vi "Folder and Path Creation.vi"(7 "Action":T1, 8 "Error In":errorcluster, 11 "Source Path for Copy":path) -> (0 "Error Out":errorcluster, 2 "Cancelled?":bool, 3 "CSV File path":path)   [LabVIEW 2012]
doc: "Generate the path to store the position save file.\nThe default position in the date folder (where the raw files are also saved)"
uses:
  Folder and Path Creation_Commands.ctl
  <vilib>/Utility/file.llb/Read From Spreadsheet File (string).vi
  <vilib>/Utility/file.llb/Write To Spreadsheet File (string).vi
  GFG/GFG library.lvlib
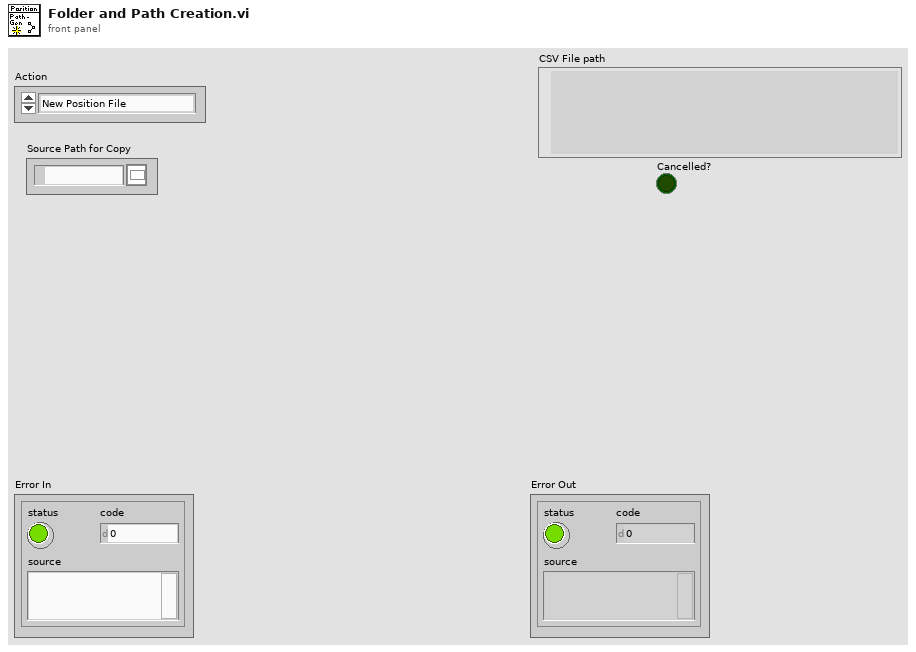
[diagram p1: front panel]
types:
  T1 = typedef "Folder and Path Creation_Commands.ctl" = enum16{"New Position File", "Load Position File", "Copy Position File"}
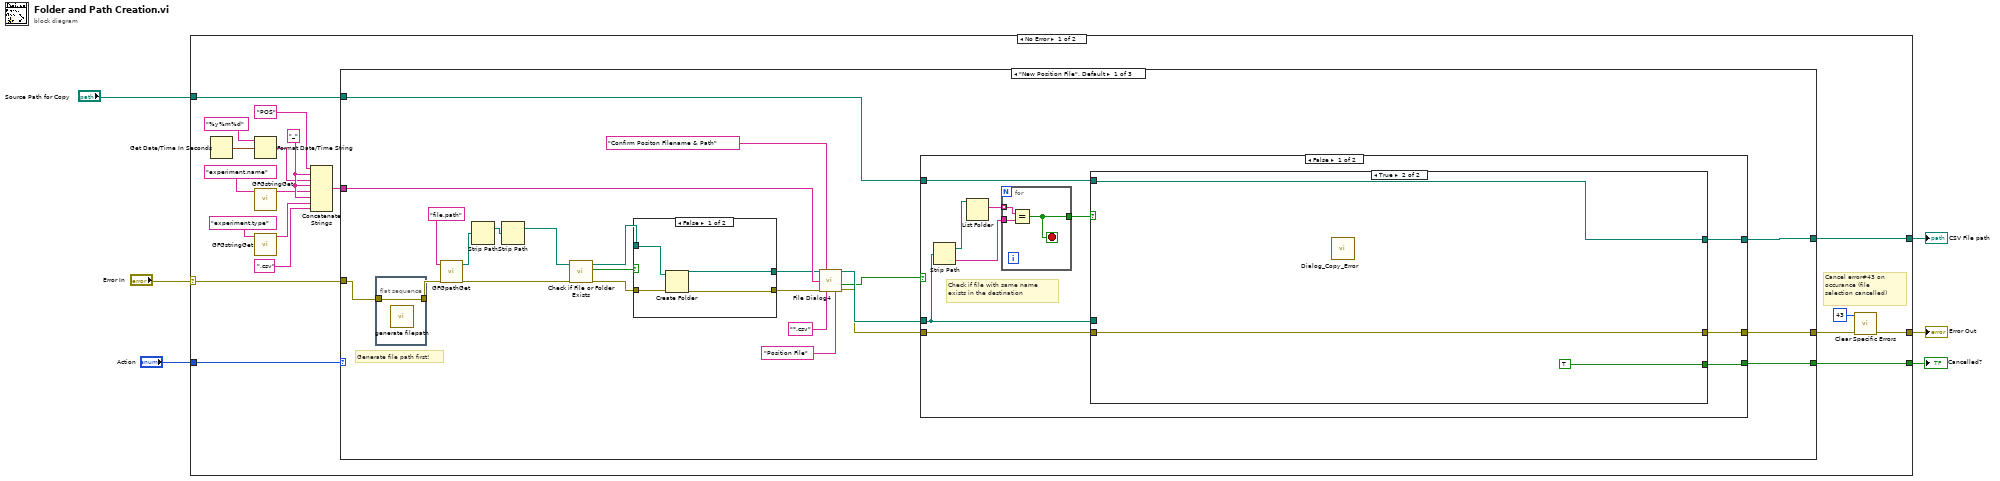
[diagram p0: block diagram]
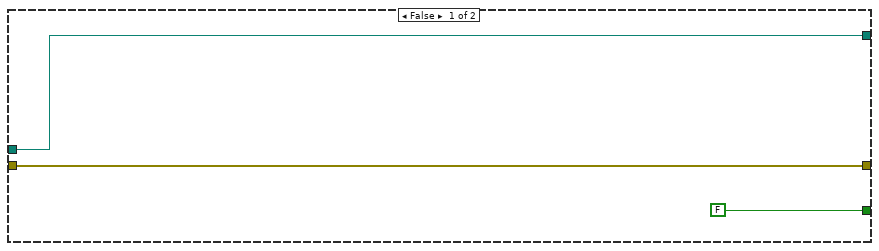
[diagram p2: hidden frame]
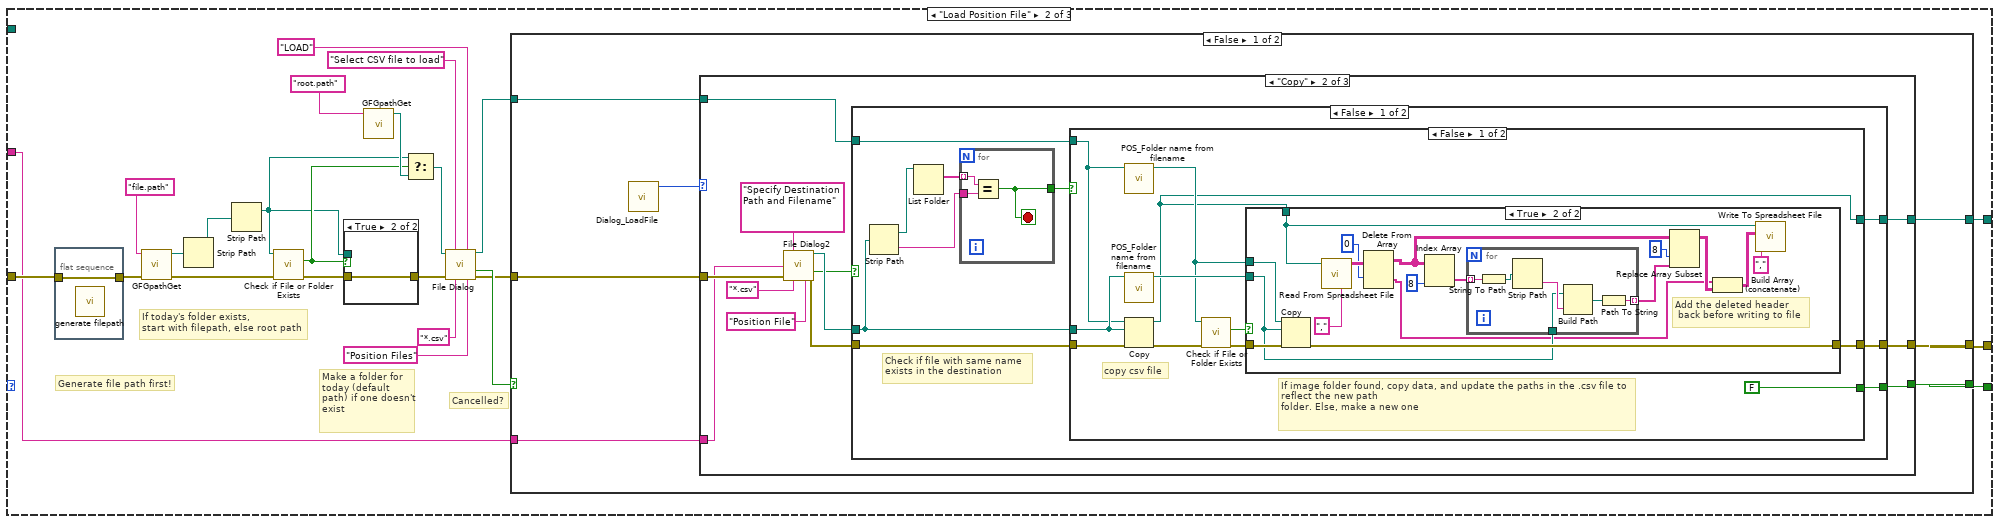
[diagram p5: hidden frame]
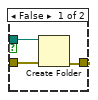
[diagram p6: hidden frame]
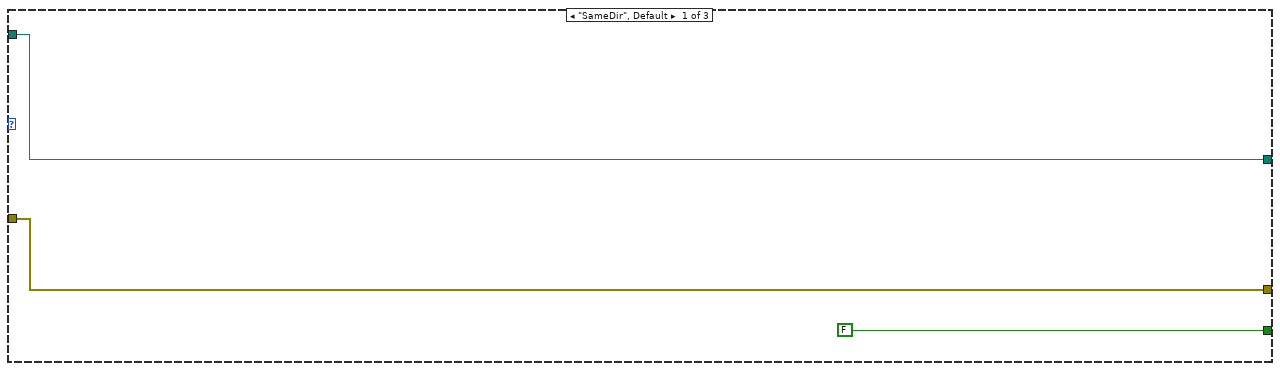
[diagram p7: hidden frame]
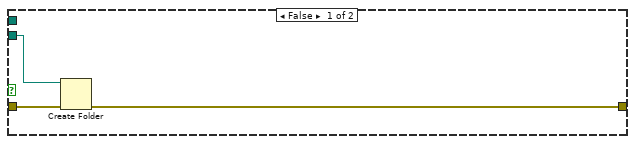
[diagram p8: hidden frame]
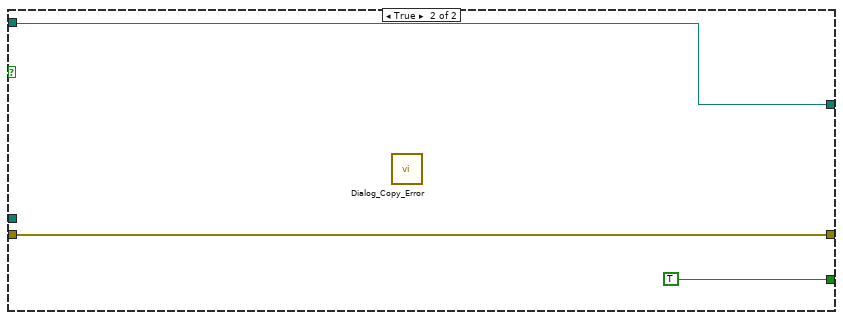
[diagram p9: hidden frame]
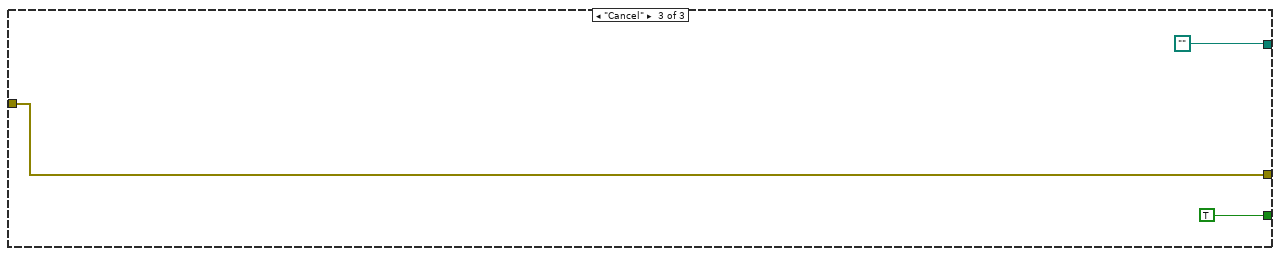
[diagram p11: hidden frame]
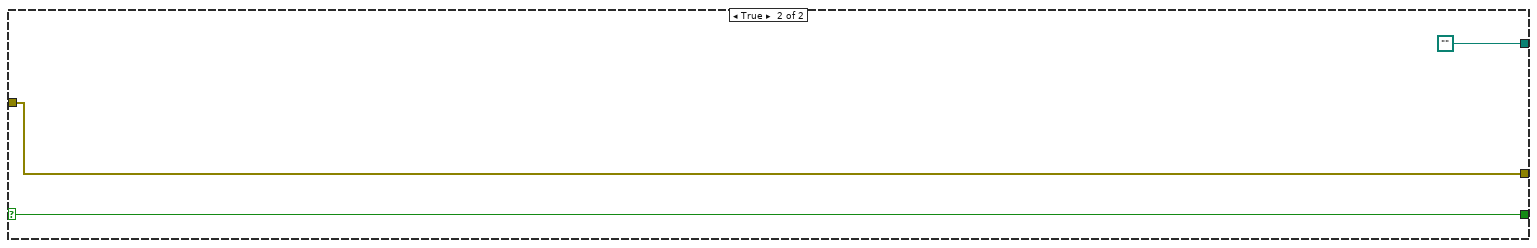
[diagram p12: hidden frame]
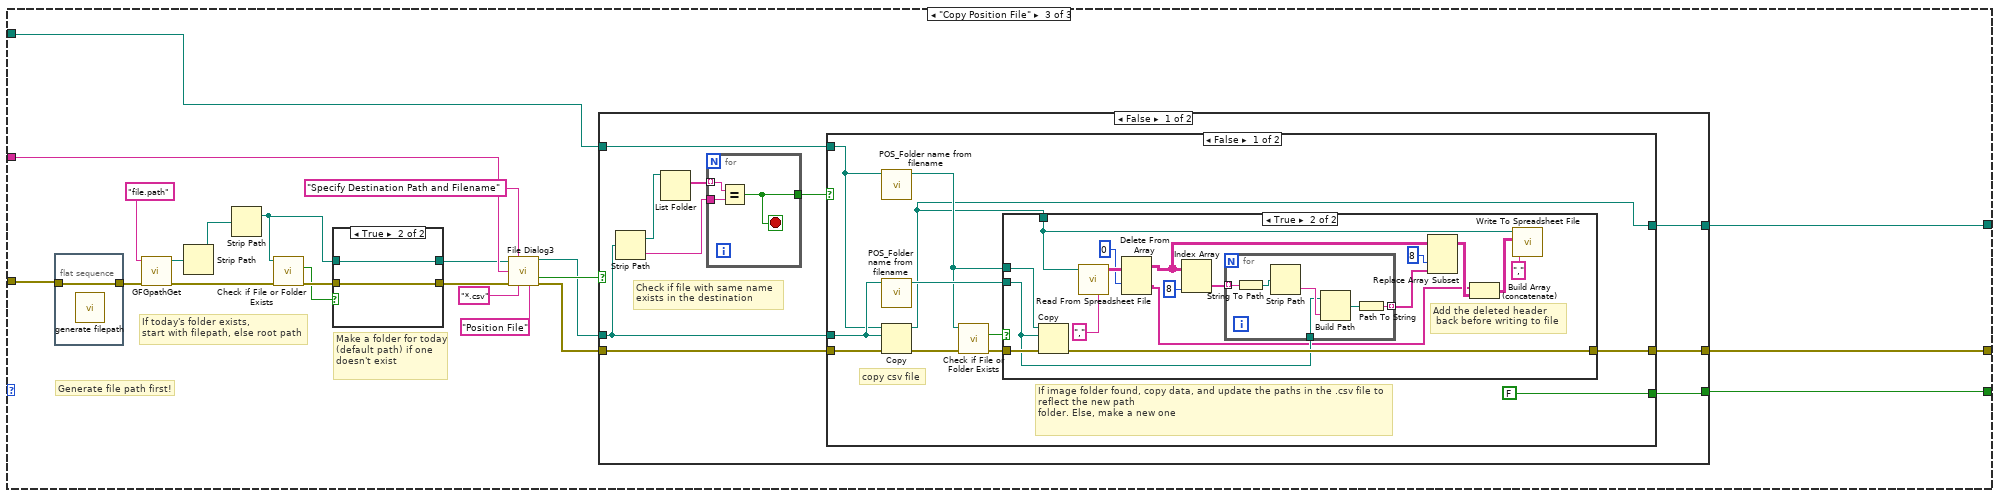
[diagram p13: hidden frame]
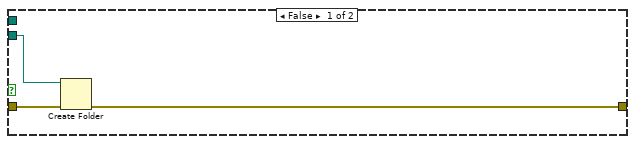
[diagram p14: hidden frame]
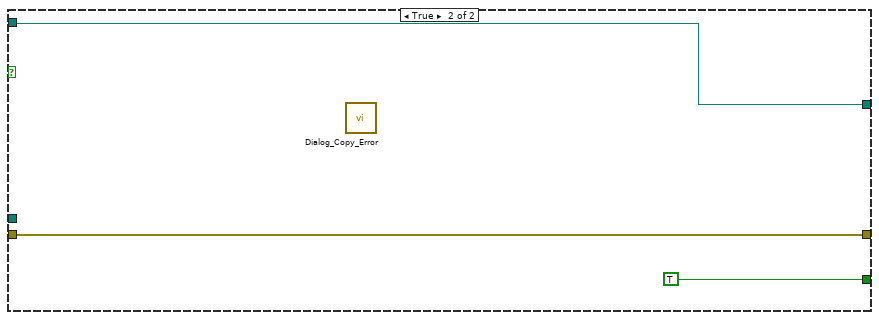
[diagram p15: hidden frame]
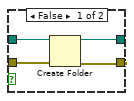
[diagram p17: hidden frame]
diagram:
  n1 = case shown="No Error" "Error In" {
    selector: "Error In" -> [w25 w276]
    tunnel: [w9 w276] -> w5
    tunnel: [w24 _] -> w4
    tunnel: "Action" -> [w23 _]
    tunnel: [w22 _] -> w2
    tunnel: "Source Path for Copy" -> [w7 _]
    frame No Error {
      w21 = "_" ("string")
      # "Cancel error#43 on occurance (file selection cancelled)"
      n2 = Get Date/Time In Seconds() -> (seconds since 1Jan1904=w14:timestamp)
      n3 = Format Date/Time String(time format string (%c)="%y%m%d", seconds (now)=w14) -> (date/time string=w17:string)  [unwired: 1 in]
      n4 = call "GFGstringGet.vi"("Variable Name in"="experiment.name") -> ("String"=w18:string)  [unwired: 10 in]
      n5 = call "GFGstringGet.vi"("Variable Name in"="experiment.type") -> ("String"=w19:string)  [unwired: 10 in]
      n6 = Concatenate Strings("POS" ("string"), w21, w17, w21, w18, w21, w19, ".csv" ("string")) -> (w12:string)
      n7 = case shown="\"New Position File\", Default" w23 {
        tunnel: [w26 w85 w195] -> w10
        tunnel: w25 -> [w40 w97 w208]
        tunnel: [w27 w86 w193] -> w24
        tunnel: [w28 w88 w194] -> w22
        tunnel: w12 -> [w38 w84 w197]
        tunnel: w7 -> [w30 _ w199]
        frame "New Position File", Default {
          # "Generate file path first!"
          n8 = flat-sequence {
            tunnel: w40 -> [w71]
            tunnel: [w71] -> w39
            frame #0 {
              n9 = call "generate filepath.vi"() -> ()  [unwired: 12 in]
            }
          }
          n10 = call "GFGpathGet.vi"("error in (no error)"=w39, "Variable Name in"="file.path") -> ("error out"=w46:errorcluster, "Path"=w47:path)  [unwired: 8 in]
          n11 = Strip Path(path=w47) -> (stripped path=w42:path)  [unwired: 1 out]
          n12 = Strip Path(path=w42) -> (stripped path=w41:path)  [unwired: 1 out]
          n13 = call <vilib>:"Check if File or Folder Exists.vi"("error in (no error)"=w46, "path"=w41) -> ("error out"=w43:errorcluster, "file or folder exists?"=w45:bool, "dup path"=w44:path)  [unwired: 7 in]
          n14 = case shown="False" w45 {
            tunnel: w44 -> [w75 w76]
            tunnel: w43 -> [w74 w77]
            tunnel: [w72 w76] -> w37
            tunnel: [w73 w77] -> w34
            frame False {
              n15 = Create Folder(path (use dialog)=w75, error in=w74) -> (created path=w72:path, error out=w73:errorcluster)  [unwired: 1 in, 1 out]
            }
            frame True {
            }
          }
          n16 = call "File Dialog4"("start path"=w37, "prompt"="Confirm Positon Filename & Path", "default name"=w38, "error in"=w34, "pattern (all files)"="*.csv", "pattern label"="Position File") -> ("selected path"=w32:path, "cancelled"=w31:bool, "error out"=w29:errorcluster)  [unwired: 6 in, 1 out]
          n17 = case shown="False" w31 {
            selector: w31 -> [_ w70]
            tunnel: [w55 w70] -> w28
            tunnel: w32 -> [w52 _]
            tunnel: w29 -> [w58 w69]
            tunnel: w30 -> [w50 w68]
            tunnel: [w56 w68] -> w27
            tunnel: [w57 w69] -> w26
            frame False {
              # "Check if file with same name\nexists in the destination"
              n18 = Strip Path(path=w52) -> (stripped path=w49:path, name=w51:string)
              n19 = List Folder(path=w49) -> (filenames=w54:string[])  [unwired: 3 in, 3 out]
              n20 = for {
                tunnel: w54 -> [w59] mode=indexing
                tunnel: [w61] -> w53
                tunnel: w51 -> [w60]
                stop <- w61 stop-if-true
                n21 = Equal?(x=w59, y=w60) -> (x = y?=w61:bool)
              }
              n22 = case shown="True" w53 {
                tunnel: w58 -> [w63 w66]
                tunnel: [w63 w66] -> w57
                tunnel: [w62 w65] -> w56
                tunnel: w50 -> [_ w65]
                tunnel: [FALSE TRUE] -> w55
                tunnel: w52 -> [w62 _]
                frame False {
                }
                frame True {
                  n23 = call "Dialog_Copy_Error.vi"() -> ()  [unwired: 12 in]
                }
              }
            }
            frame True {
            }
          }
        }
        frame "Load Position File" {
          # "Make a folder for today (default\npath) if one doesn't exist"
          # "If today's folder exists,\nstart with filepath, else root path"
          # "Cancelled?"
          # "Generate file path first!"
          n24 = flat-sequence {
            tunnel: w97 -> [w190]
            tunnel: [w190] -> w96
            frame #0 {
              n25 = call "generate filepath.vi"() -> ()  [unwired: 12 in]
            }
          }
          n26 = call "GFGpathGet.vi"("error in (no error)"=w96, "Variable Name in"="file.path") -> ("error out"=w99:errorcluster, "Path"=w100:path)  [unwired: 8 in]
          n27 = Strip Path(path=w100) -> (stripped path=w98:path)  [unwired: 1 out]
          n28 = Strip Path(path=w98) -> (stripped path=w80:path)  [unwired: 1 out]
          n29 = call <vilib>:"Check if File or Folder Exists.vi"("error in (no error)"=w99, "path"=w80) -> ("error out"=w83:errorcluster, "file or folder exists?"=w81:bool)  [unwired: 7 in, 1 out]
          n30 = case shown="True" w81 {
            tunnel: w80 -> [w104 _]
            tunnel: w83 -> [w103 w105]
            tunnel: [w102 w105] -> w82
            frame False {
              n31 = Create Folder(path (use dialog)=w104, error in=w103) -> (error out=w102:errorcluster)  [unwired: 1 in, 2 out]
            }
            frame True {
            }
          }
          n32 = call "GFGpathGet.vi"("Variable Name in"="root.path") -> ("Path"=w94:path)  [unwired: 9 in, 1 out]
          n33 = Select(t=w80, s=w81, f=w94) -> (s? t:f=w93:path)
          n34 = call "File Dialog"("start path"=w93, "prompt"="Select CSV file to load", "button label"="LOAD", "error in"=w82, "pattern (all files)"="*.csv", "pattern label"="Position Files") -> ("selected path"=w89:path, "cancelled"=w92:bool, "error out"=w91:errorcluster)  [unwired: 6 in, 1 out]
          n35 = case shown="False" w92 {
            selector: w92 -> [_ w189]
            tunnel: w91 -> [w110 w187]
            tunnel: w89 -> [w111 _]
            tunnel: [w112 w189] -> w88
            tunnel: [w109 path ""] -> w86
            tunnel: [w108 w187] -> w85
            tunnel: w84 -> [w107 _]
            frame False {
              n36 = call "Dialog_LoadFile.vi"() -> ("LoadAction OUT"=w106:enum32{"SameDir", "Copy", "Cancel"})  [unwired: 11 in]
              n37 = case shown="\"Copy\"" w106 {
                tunnel: [FALSE w120 TRUE] -> w112
                tunnel: w111 -> [w115 w118 _]
                tunnel: w110 -> [w114 w122 w185]
                tunnel: [w115 w119 path ""] -> w109
                tunnel: [w114 w121 w185] -> w108
                tunnel: w107 -> [_ w116 _]
                frame "SameDir", Default {
                }
                frame "Copy" {
                  n38 = call "File Dialog2"("prompt"="Specify Destination Path and Filename", "default name"=w116, "error in"=w122, "pattern (all files)"="*.csv", "pattern label"="Position File") -> ("selected path"=w127:path, "cancelled"=w125:bool, "error out"=w126:errorcluster)  [unwired: 7 in, 1 out]
                  n39 = case shown="False" w125 {
                    selector: w125 -> [_ w183]
                    tunnel: [w134 w183] -> w120
                    tunnel: w127 -> [w131 _]
                    tunnel: w126 -> [w137 w182]
                    tunnel: w118 -> [w129 w181]
                    tunnel: [w135 w181] -> w119
                    tunnel: [w136 w182] -> w121
                    frame False {
                      # "Check if file with same name\nexists in the destination"
                      n40 = Strip Path(path=w131) -> (stripped path=w128:path, name=w130:string)
                      n41 = List Folder(path=w128) -> (filenames=w133:string[])  [unwired: 3 in, 3 out]
                      n42 = for {
                        tunnel: w133 -> [w138] mode=indexing
                        tunnel: [w140] -> w132
                        tunnel: w130 -> [w139]
                        stop <- w140 stop-if-true
                        n43 = Equal?(x=w138, y=w139) -> (x = y?=w140:bool)
                      }
                      n44 = case shown="False" w132 {
                        tunnel: w137 -> [w151 w179]
                        tunnel: [w150 w179] -> w136
                        tunnel: [w143 w178] -> w135
                        tunnel: w129 -> [w141 w178]
                        tunnel: [FALSE TRUE] -> w134
                        tunnel: w131 -> [w142 _]
                        frame False {
                          # "If image folder found, copy data, and update the paths in the .csv file to reflect the new path\nfolder. Else, make a new one"
                          # "copy csv file"
                          n45 = call "POS_Folder name from filename.vi"("File Path In"=w141) -> ("Folder Path Out"=w145:path)  [unwired: 10 in]
                          n46 = call "POS_Folder name from filename.vi"("File Path In"=w142) -> ("Folder Path Out"=w146:path)  [unwired: 10 in]
                          n47 = Copy(8:w151, 10:w142, 11:w141) -> (0:w149:errorcluster, 3:w143:path)  [unwired: 2 in, 1 out]
                          n48 = call <vilib>:"Check if File or Folder Exists.vi"("error in (no error)"=w149, "path"=w145) -> ("error out"=w148:errorcluster, "file or folder exists?"=w147:bool)  [unwired: 7 in, 1 out]
                          n49 = case shown="True" w147 {
                            tunnel: [w154 w171] -> w150
                            tunnel: w148 -> [w153 w170]
                            tunnel: w145 -> [_ w169]
                            tunnel: w146 -> [w152 w165]
                            tunnel: w143 -> [_ w162]
                            frame False {
                              n50 = Create Folder(path (use dialog)=w152, error in=w153) -> (error out=w154:errorcluster)  [unwired: 1 in, 2 out]
                            }
                            frame True {
                              # "Add the deleted header\n back before writing to file"
                              n51 = Copy(8:w170, 10:w165, 11:w169) -> (0:w171:errorcluster)  [unwired: 2 in, 2 out]
                              n52 = call-poly <vilib>:"Read From Spreadsheet File.vi"("delimiter (\\t)"="," ("delimiter (\\t)"), "file path (dialog if empty)"=w162) -> ("all rows"=w158:string[][])  [unwired: 5 in, 4 out]
                              n53 = Delete From Array(array=w158, index (row)=0) -> (deleted portion=w155:string[], array with subset deleted=w157:string[][])  [unwired: 2 in]
                              n54 = Index Array(array=w157, index (col)=8 ("disabled index (col)")) -> (element=w166:string[])  [unwired: 1 in]
                              n55 = for {
                                tunnel: w166 -> [w177] mode=indexing
                                tunnel: w165 -> [w174]
                                tunnel: [w172] -> w163 mode=indexing
                                n56 = String To Path(string=w177) -> (path=w176:path)
                                n57 = Strip Path(path=w176) -> (name=w175:string)  [unwired: 1 out]
                                n58 = Build Path(base path=w174, name or relative path=w175) -> (appended path=w173:path)
                                n59 = Path To String(path=w173) -> (string=w172:string)
                              }
                              n60 = Replace Array Subset(array=w157, new element=w163, index (col)=8 ("disabled index (col)")) -> (w160:string[][])  [unwired: 1 in]
                              n61 = Build Array (concatenate)(w155, w160) -> (w159:string[][])
                              n62 = call-poly <vilib>:"Write To Spreadsheet File.vi"("delimiter (\\t)"="," ("delimiter (\\t)"), "2D data"=w159, "file path (dialog if empty)"=w162) -> ()  [unwired: 5 in, 1 out]
                            }
                          }
                        }
                        frame True {
                          n63 = call "Dialog_Copy_Error.vi"() -> ()  [unwired: 12 in]
                        }
                      }
                    }
                    frame True {
                    }
                  }
                }
                frame "Cancel" {
                }
              }
            }
            frame True {
            }
          }
        }
        frame "Copy Position File" {
          # "Make a folder for today (default path) if one doesn't exist"
          # "If today's folder exists,\nstart with filepath, else root path"
          # "Generate file path first!"
          n64 = flat-sequence {
            tunnel: w208 -> [w275]
            tunnel: [w275] -> w207
            frame #0 {
              n65 = call "generate filepath.vi"() -> ()  [unwired: 12 in]
            }
          }
          n66 = call "GFGpathGet.vi"("error in (no error)"=w207, "Variable Name in"="file.path") -> ("error out"=w210:errorcluster, "Path"=w211:path)  [unwired: 8 in]
          n67 = Strip Path(path=w211) -> (stripped path=w209:path)  [unwired: 1 out]
          n68 = Strip Path(path=w209) -> (stripped path=w204:path)  [unwired: 1 out]
          n69 = call <vilib>:"Check if File or Folder Exists.vi"("error in (no error)"=w210, "path"=w204) -> ("error out"=w206:errorcluster, "file or folder exists?"=w205:bool)  [unwired: 7 in, 1 out]
          n70 = case shown="True" w205 {
            tunnel: w204 -> [w272 w273]
            tunnel: w206 -> [w271 w274]
            tunnel: [w270 w274] -> w198
            tunnel: [w269 w273] -> w196
            frame False {
              n71 = Create Folder(path (use dialog)=w272, error in=w271) -> (created path=w269:path, error out=w270:errorcluster)  [unwired: 1 in, 1 out]
            }
            frame True {
            }
          }
          n72 = call "File Dialog3"("start path"=w196, "prompt"="Specify Destination Path and Filename", "default name"=w197, "error in"=w198, "pattern (all files)"="*.csv", "pattern label"="Position File") -> ("selected path"=w201:path, "cancelled"=w202:bool, "error out"=w200:errorcluster)  [unwired: 6 in, 1 out]
          n73 = case shown="False" w202 {
            selector: w202 -> [_ w268]
            tunnel: [w219 w268] -> w194
            tunnel: w201 -> [w216 _]
            tunnel: w200 -> [w222 w267]
            tunnel: w199 -> [w214 w266]
            tunnel: [w220 w266] -> w193
            tunnel: [w221 w267] -> w195
            frame False {
              # "Check if file with same name\nexists in the destination"
              n74 = Strip Path(path=w216) -> (stripped path=w213:path, name=w215:string)
              n75 = List Folder(path=w213) -> (filenames=w218:string[])  [unwired: 3 in, 3 out]
              n76 = for {
                tunnel: w218 -> [w223] mode=indexing
                tunnel: [w225] -> w217
                tunnel: w215 -> [w224]
                stop <- w225 stop-if-true
                n77 = Equal?(x=w223, y=w224) -> (x = y?=w225:bool)
              }
              n78 = case shown="False" w217 {
                tunnel: w222 -> [w236 w264]
                tunnel: [w235 w264] -> w221
                tunnel: [w228 w263] -> w220
                tunnel: w214 -> [w226 w263]
                tunnel: [FALSE TRUE] -> w219
                tunnel: w216 -> [w227 _]
                frame False {
                  # "If image folder found, copy data, and update the paths in the .csv file to reflect the new path\nfolder. Else, make a new one"
                  # "copy csv file"
                  n79 = call "POS_Folder name from filename.vi"("File Path In"=w226) -> ("Folder Path Out"=w230:path)  [unwired: 10 in]
                  n80 = call "POS_Folder name from filename.vi"("File Path In"=w227) -> ("Folder Path Out"=w231:path)  [unwired: 10 in]
                  n81 = Copy(8:w236, 10:w227, 11:w226) -> (0:w234:errorcluster, 3:w228:path)  [unwired: 2 in, 1 out]
                  n82 = call <vilib>:"Check if File or Folder Exists.vi"("error in (no error)"=w234, "path"=w230) -> ("error out"=w233:errorcluster, "file or folder exists?"=w232:bool)  [unwired: 7 in, 1 out]
                  n83 = case shown="True" w232 {
                    tunnel: [w239 w256] -> w235
                    tunnel: w233 -> [w238 w255]
                    tunnel: w230 -> [_ w254]
                    tunnel: w231 -> [w237 w250]
                    tunnel: w228 -> [_ w247]
                    frame False {
                      n84 = Create Folder(path (use dialog)=w237, error in=w238) -> (error out=w239:errorcluster)  [unwired: 1 in, 2 out]
                    }
                    frame True {
                      # "Add the deleted header\n back before writing to file"
                      n85 = Copy(8:w255, 10:w250, 11:w254) -> (0:w256:errorcluster)  [unwired: 2 in, 2 out]
                      n86 = call-poly <vilib>:"Read From Spreadsheet File.vi"("delimiter (\\t)"="," ("delimiter (\\t)"), "file path (dialog if empty)"=w247) -> ("all rows"=w243:string[][])  [unwired: 5 in, 4 out]
                      n87 = Delete From Array(array=w243, index (row)=0) -> (deleted portion=w240:string[], array with subset deleted=w242:string[][])  [unwired: 2 in]
                      n88 = Index Array(array=w242, index (col)=8 ("disabled index (col)")) -> (element=w251:string[])  [unwired: 1 in]
                      n89 = for {
                        tunnel: w251 -> [w262] mode=indexing
                        tunnel: w250 -> [w259]
                        tunnel: [w257] -> w248 mode=indexing
                        n90 = String To Path(string=w262) -> (path=w261:path)
                        n91 = Strip Path(path=w261) -> (name=w260:string)  [unwired: 1 out]
                        n92 = Build Path(base path=w259, name or relative path=w260) -> (appended path=w258:path)
                        n93 = Path To String(path=w258) -> (string=w257:string)
                      }
                      n94 = Replace Array Subset(array=w242, new element=w248, index (col)=8 ("disabled index (col)")) -> (w245:string[][])  [unwired: 1 in]
                      n95 = Build Array (concatenate)(w240, w245) -> (w244:string[][])
                      n96 = call-poly <vilib>:"Write To Spreadsheet File.vi"("delimiter (\\t)"="," ("delimiter (\\t)"), "2D data"=w244, "file path (dialog if empty)"=w247) -> ()  [unwired: 5 in, 1 out]
                    }
                  }
                }
                frame True {
                  n97 = call "Dialog_Copy_Error.vi"() -> ()  [unwired: 12 in]
                }
              }
            }
            frame True {
            }
          }
        }
      }
      n98 = call "Clear Specific Errors.vi"("Error In"=w10, "Error number In"=43) -> ("Error Out"=w9:errorcluster)  [unwired: 8 in, 1 out]
    }
    frame Error {
    }
  }
  "Error Out" <- w5
  "CSV File path" <- w4
  "Cancelled?" <- w2
